vi "Finalize Turn.vi"(6 "Turn Results In":T1, 8 "error in (no error)":errorcluster, 11 "Map in":refnum<class "Map.lvclass">) -> (0 "error out":errorcluster, 3 "Map out":refnum<class "Map.lvclass">, 4 "Turn Results":T1)   [LabVIEW 2020, in "SquareBattle.lvlib" / "Map.lvclass"]
uses:
  Map.lvclass
  Turn Results.ctl
  Map.lvclass/Map.ctl
  SquareBattle.lvlib
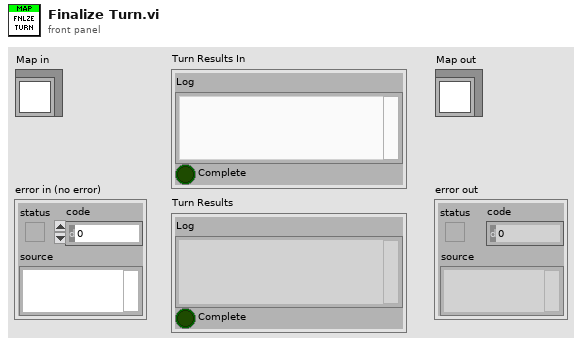
[diagram p1: front panel]
types:
  T1 = typedef "SquareBattle.lvlib/Turn Results.ctl" = cluster{"Log":string, "Complete":bool}
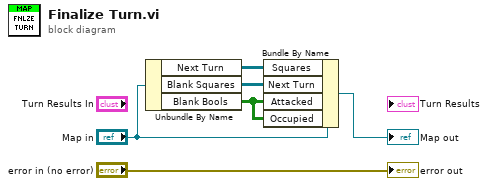
[diagram p0: block diagram]
diagram:
  n1 = Unbundle By Name("Map in") -> ("Next Turn"=w5:refnum<class "Square.lvclass">[][], "Blank Squares"=w4:refnum<class "Square.lvclass">[][], "Blank Bools"=w3:bool[][])
  n2 = Bundle By Name(cluster="Map in", "Squares"=w5, "Next Turn"=w4, "Attacked"=w3, "Occupied"=w3) -> (→"Map out":refnum<class "Map.lvclass">)
  "error out" <- "error in (no error)"
